vi "Periodic Tasks.vi"(8 "error in (no error)":errorcluster) -> (0 "error out":errorcluster)   [LabVIEW 2020]
doc: "This VI runs in parallel to other tasks. It can contain as many user-defined periodic loops as you need. These can carry out PID or other sorts of timed response."
uses:
  Robot Global Data.vi
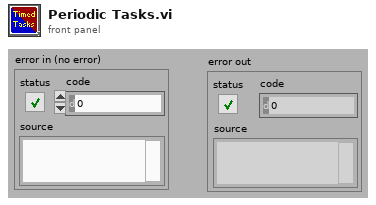
[diagram p1: front panel]
types:
  T1 = typedef "WPI_DriverStationRobotMode2.ctl" = enum16{"Autonomous Disabled", "Autonomous Enabled", "Teleop Disabled", "Teleop Enabled", "Disconnected", "Finish", "Test Disabled", "Test Enabled", "Emergency Stopped"}
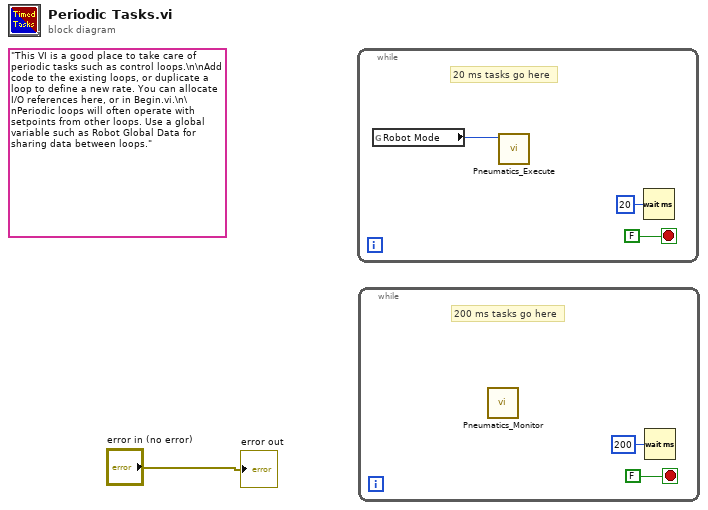
[diagram p0: block diagram]
diagram:
  (unwired) "This VI is a good place to take care of periodic tasks such as control loops.\n\nAdd code to the existing loops, or duplicate a loop to define a new rate. You can allocate I/O references here, or in Begin.vi.\n\nPeriodic loops will often operate with setpoints from other loops. Use a global variable such as Robot Global Data for sharing data between loops."
  n1 = while {
    stop <- FALSE stop-if-true
    # "20 ms tasks go here"
    n2 = global read "Robot Global Data.vi" "Robot Mode"() -> (w2:T1)
    n3 = call "Pneumatics_Execute.vi"("Robot Mode"=w2) -> ()  [unwired: 10 in, 1 out]
    n4 = Wait (ms)(milliseconds to wait=u32 20) -> ()  [unwired: 1 out]
  }
  n5 = while {
    stop <- FALSE stop-if-true
    # "200 ms tasks go here"
    n6 = call "Pneumatics_Monitor.vi"() -> ()  [unwired: 11 in, 1 out]
    n7 = Wait (ms)(milliseconds to wait=u32 200) -> ()  [unwired: 1 out]
  }
  "error out" <- "error in (no error)"
